vi "Teleop.vi"(10 "Match Info":T1={"Autonomous Elapsed Seconds"=0.0, "TeleOp Elapsed Seconds"=0.0, "Disabled Elapsed Seconds"=0.0, "Visited Autonomous"=FALSE, "Visited TeleOp"=FALSE, "Visited Disabled"=FALSE, "Autonomous Settings"={"Autonomous Style"=enum."Independent", "VI Refnum"=refnum}}, 11 "Call Context":T2) -> ()   [LabVIEW 2016]
doc: "This VI is called for each TeleOp packet received from the DS where the robot is not disabled. It is often used to read from the joysticks and update I/O or to update setpoints for timed control loops. It should complete and return within 20 milliseconds or it may miss DS packets."
uses:
  <vilib>/Rock Robotics/WPI/DriverStation/WPI_DriverStationDerivedRobotMode.ctl
  <vilib>/Rock Robotics/WPI/DriverStation/WPI_DriverStationMatch Info.ctl
  <vilib>/Rock Robotics/WPI/ThirdParty/CanMotor/TalonSRX/WPI_CANTalonSRX_APIFeedbackSelect.ctl
  <vilib>/Rock Robotics/WPI/ThirdParty/CanMotor/TalonSRX/WPI_CANTalonSRX_Params.ctl
  <vilib>/Rock Robotics/WPI/ThirdParty/CanMotor/TalonSRX/WPI_CANTalonSRX_APIControlMode.ctl
  <vilib>/Rock Robotics/WPI/Utilities/WPI_GetSetVariantRefNum.vi
panel:
  out "SensorPos (rotations)":dbl
  out "Motor output Plot":cluster{"Applied Throttle":dbl}(graph)
  out "Target Position (rotations)":dbl
  out "SensorRPM Velocity RPM":dbl
  in  "Ramp Rate":dbl
  in  "I Zone":dbl
  in  "F - Generally is zero for position-servo":dbl
  in  "D":dbl
  in  "I":dbl
  in  "P":dbl
  out "Applied Output":dbl
  out "Position Closed Loop Plots":cluster{dbl, "Sensor Velocity":dbl}(graph)
  # "Press and Hold Button1 to drive Talon directly.  Make sure sensor position moves in positive direction when Talon LEDs are green.\n\nMomentary press Button2 to activate Position closed-loop.  The gamepad y-axis is sampled once and scaled to provide a target set point.\n\nPress Button3 to \"zero\" the sensor position.\n\nPress Button4 to \"seed\" the Sensor position with the Absolute Position reported by the CTRE Magnetic Encoder."
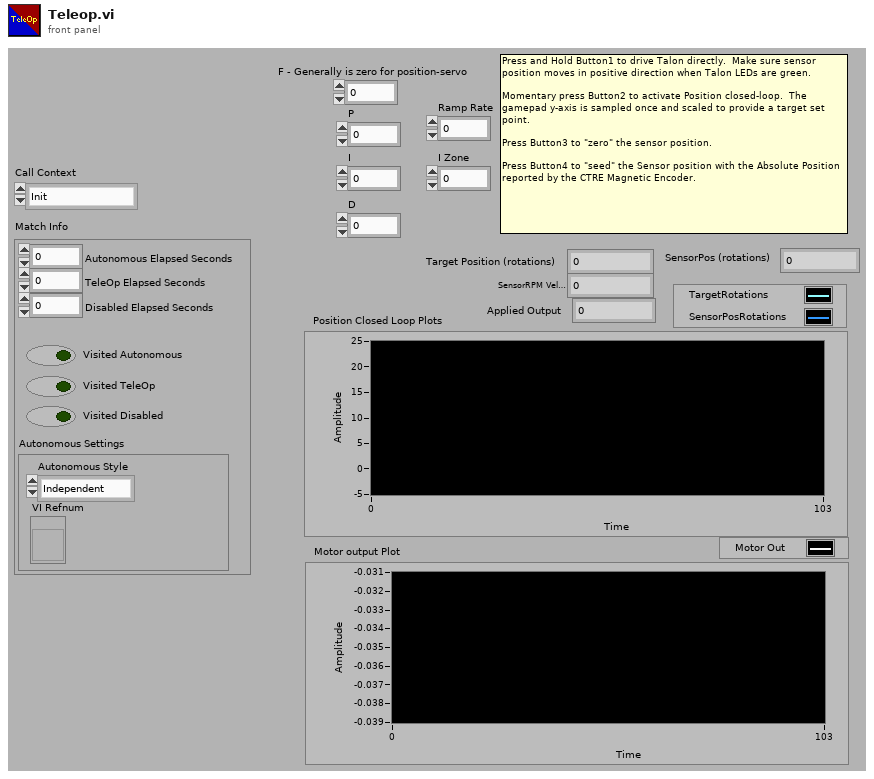
[diagram p1: front panel]
types:
  T1 = typedef "WPI_DriverStationMatch Info.ctl" = cluster{"Autonomous Elapsed Seconds":dbl, "TeleOp Elapsed Seconds":dbl, "Disabled Elapsed Seconds":dbl, "Visited Autonomous":bool, "Visited TeleOp":bool, "Visited Disabled":bool, "Autonomous Settings":cluster{"Autonomous Style":enum16{"Iterative", "Independent"}, "VI Refnum":refnum<vi>}}
  T2 = typedef "WPI_DriverStationDerivedRobotMode.ctl" = enum16{"Init", "Execute", "Stop"}
  T3 = typedef "WPI_CANTalonSRX_APIFeedbackSelect.ctl" = enum16{"Digital Quadrature Encoder", "Analog Potentiometer", "Analog Encoder", "Count on Quad-A (Rising-Edge)", "Count on Quad-A (Falling-Edge)", "CTR Magnetic Enc (Absolute)", "CTR Magnetic Enc (Relative)", "Pulse Width"}
  T4 = typedef "WPI_JoystickDevRef.ctl" = cluster{"Device":T5}
  T5 = typedef "WPI_JoystickDeviceEnum.ctl" = enum16{"USB 0", "USB 1", "USB 2", "USB 3", "USB 4", "USB 5"}
  T6 = typedef "WPI_MotorControlDeviceRef.ctl" = cluster{"DeviceStatus":errorcluster, "Type":T7, "PWM":cluster{"PWM Channel":T8, "DeadBand":T9}, "CAN":cluster{"Device Number":u8, "SetOutput VI Ref":variant, "GetOutput VI Ref":variant, "Enable VI Ref":variant, "Disable VI Ref":variant, "Data":variant}, "Invert":bool}
  T7 = typedef "WPI_MotorControlType.ctl" = enum16{"PWM", "CAN"}
  T8 = typedef "FPGA_DIOPWMChannel.ctl" = enum8{"PWM 0", "PWM 1", "PWM 2", "PWM 3", "PWM 4", "PWM 5", "PWM 6", "PWM 7", "PWM 8", "PWM 9", "PWM MXP 0", "PWM MXP 1", "PWM MXP 2", "PWM MXP 3", "PWM MXP 4", "PWM MXP 5", "PWM MXP 6", "PWM MXP 7", "PWM MXP 8", "PWM MXP 9", "Invalid"}
  T9 = typedef "WPI_PWMDeadband.ctl" = cluster{"Name":string, "maxPositivePwm":i32, "minPositivePwm":i32, "centerPwm":i32, "maxNegativePwm":i32, "minNegativePwm":i32, "angularRange":u16}
  T10 = typedef "WPI_CANTalonSRX_APIControlMode.ctl" = enum8{"Percent VBus", "Speed", "Position", "Slave", "Unchanged / Invalid", "Voltage Compensation", "Current", "Motion Profile", "Motion Magic"}
  T11 = typedef "WPI_CANTalonSRX_Params.ctl" = u8
  T12 = typedef "WPI_CANTalonSRX_GlobalStatus.ctl" = cluster{"Applied Throttle":dbl, "Module Enabled":bool, "CAN Error":errorcluster, "Closed Loop Error":dbl, "Forward Limit Switch Closed":bool, "Reverse Limit Switch Closed":bool, "Sensor Position":dbl, "Sensor Velocity":dbl, "Current":dbl, "Sticky Fault - Over Temp":bool, "Sticky Fault - Under Voltage":bool, "Sticky Fault - Forward Limit":bool, "Sticky Fault - Reverse Limit":bool, "Sticky Fault - Forward Soft Limit":bool, "Sticky Fault - Reverse Soft Limit":bool, "Brake is Enabled":bool, "Encoder Position":dbl, "Encoder Velocity":dbl, "Encoder Index Count":dbl, "Encoder A Pin State":bool, "Encoder B Pin State":bool, "Encoder Index Pin State":bool, "Analog In":dbl, "Analog In Velocity":dbl, "Temperature (C)":dbl, "Battery Voltage":dbl, "Control 5 Is Supported":bool, "Current Profile Slot Select":dbl, "Pos Div 8":bool, "Vel Div 4":bool, "Pulse Width Position":i32, "Pulse Width Velocity":i32, "Pulse Width Rise To Rise (us)":i32, "Pulse Width Rise To Fall (us)":i32, "Mot Prof Active Is Under Run":bool, "Mot Prof Active Has Under Run":bool, "Mot Prof Active Is Last":bool, "Mot Prof Active Velocity Only":bool, "Mot Prof Active Is Valid":bool, "Mot Prof Buffer Is Full":bool, "Mot Prof Active Profile Slot Select":i32, "Mot Prof NextID":i32, "Mot Prof Count":i32, "Mot Prof Active Velocity":dbl, "Mot Prof Active Position":dbl, "Mot Prof Output Enable":i32}
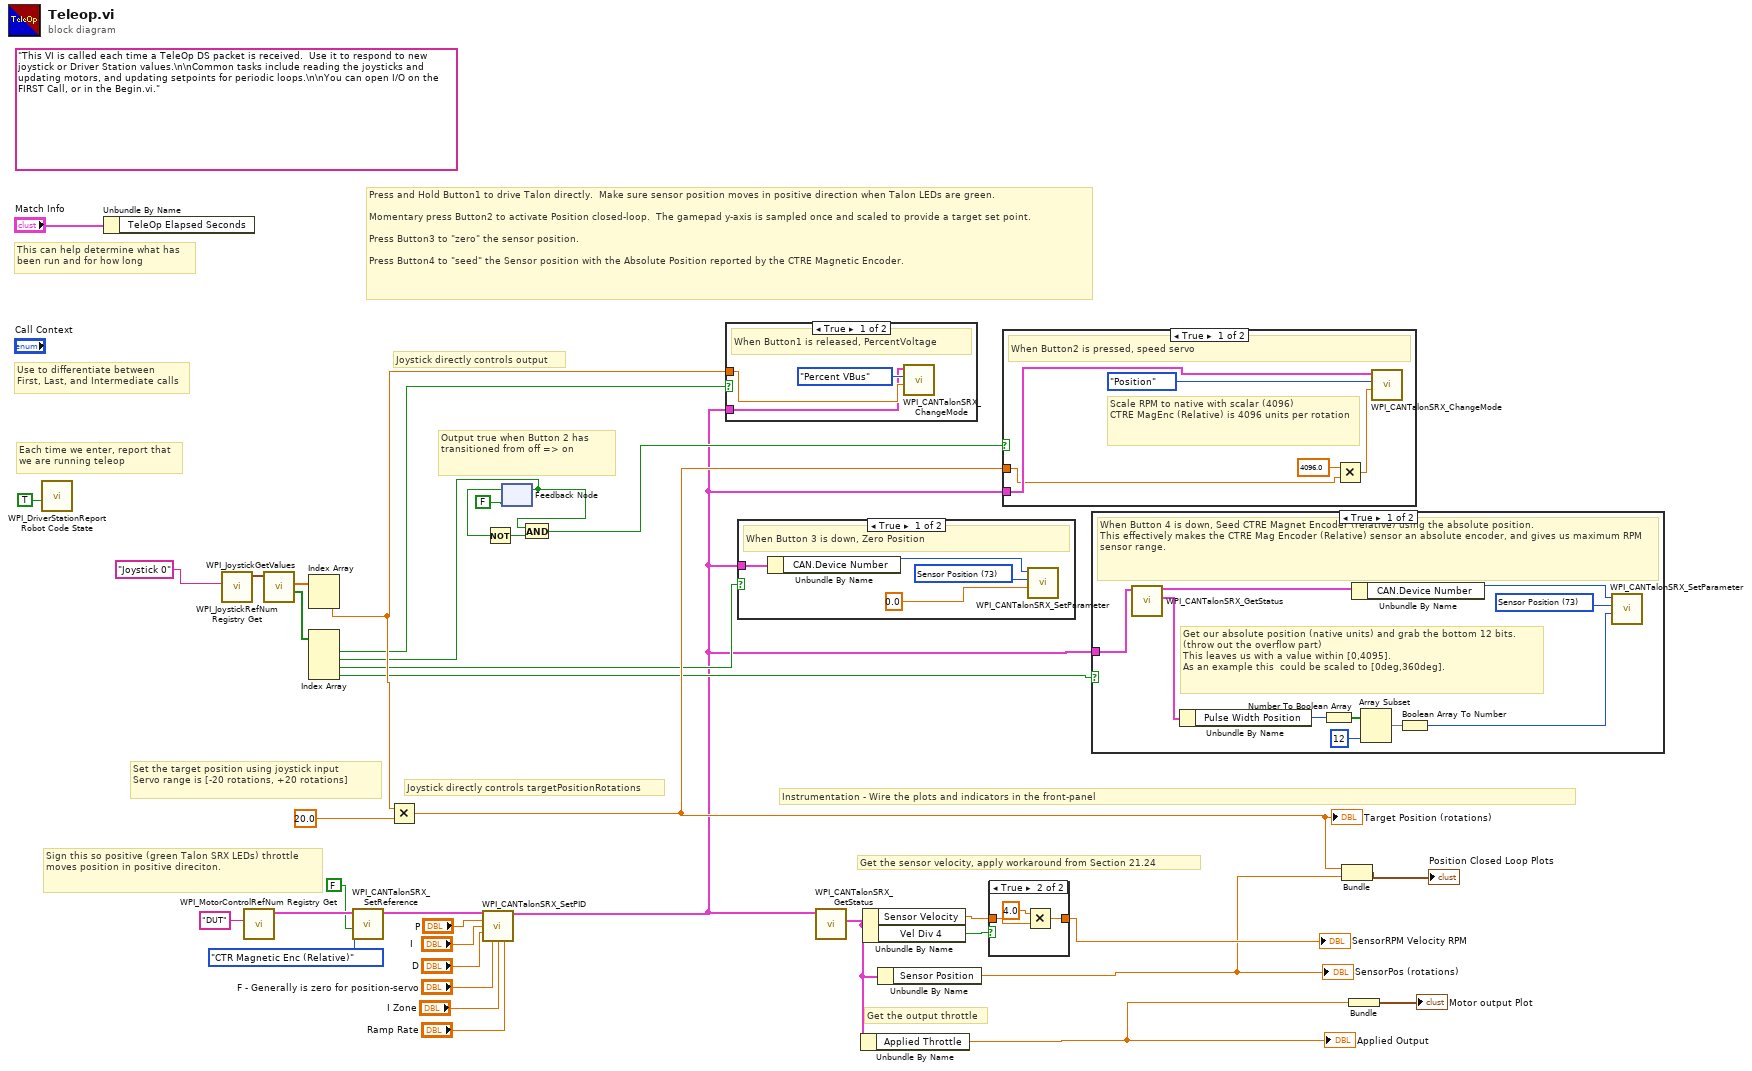
[diagram p0: block diagram]
diagram:
  (unwired) "This VI is called each time a TeleOp DS packet is received.  Use it to respond to new joystick or Driver Station values.\n\nCommon tasks include reading the joysticks and updating motors, and updating setpoints for periodic loops.\n\nYou can open I/O on the FIRST Call, or in the Begin.vi."
  # "Sign this so positive (green Talon SRX LEDs) throttle moves position in positive direciton."
  # "Instrumentation - Wire the plots and indicators in the front-panel"
  # "Output true when Button 2 has transitioned from off => on"
  # "Press and Hold Button1 to drive Talon directly.  Make sure sensor position moves in positive direction when Talon LEDs are green.\n\nMomentary press Button2 to activate Position closed-loop.  The gamepad y-axis is sampled once and scaled to provide a target set point.\n\nPress Button3 to \"zero\" the sensor position.\n\nPress Button4 to \"seed\" the Sensor position with the Absolute Position reported by the CTRE Magnetic Encoder."
  # "Get the output throttle"
  # "Get the sensor velocity, apply workaround from Section 21.24"
  # "Joystick directly controls targetPositionRotations"
  # "Joystick directly controls output"
  # "Set the target position using joystick input\nServo range is [-20 rotations, +20 rotations]"
  # "Each time we enter, report that\nwe are running teleop"
  # "Use to differentiate between\nFirst, Last, and Intermediate calls"
  # "This can help determine what has\nbeen run and for how long"
  n1 = call <vilib>:"WPI_DriverStationReport Robot Code State.vi"("TeleOp"=TRUE ("Autonomous")) -> ()  [unwired: 10 in, 1 out]
  n2 = Unbundle By Name("Match Info") -> ()  [unwired: 1 out]
  n3 = call <vilib>:"WPI_JoystickRefNum Registry Get.vi"("refnum name"="Joystick 0") -> ("JoystickDevRef"=w35:T4)  [unwired: 1 in, 9 out]
  n4 = call <vilib>:"WPI_MotorControlRefNum Registry Get.vi"("refnum name"="DUT") -> ("MotorControlDevRef"=w19:T6)  [unwired: 9 in, 1 out]
  n5 = call <vilib>:"WPI_JoystickGetValues.vi"("JoystickDevRef"=w35) -> ("Buttons"=w32:bool[], "Axes"=w33:dbl[])  [unwired: 6 in, 3 out]
  n6 = Index Array(array=w33) -> (element #2=w12:dbl)  [unwired: 2 in, 1 out]
  n7 = Index Array(array=w32) -> (element #1=w9:bool, element #2=w7:bool, element #3=w5:bool, element #4=w3:bool)  [unwired: 4 in]
  n8 = call <vilib>:"WPI_CANTalonSRX_SetReference.vi"("Reverse Feedback Sensor"=FALSE, "Feedback Reference"=WPI_CANTalonSRX_APIFeedbackSelect."CTR Magnetic Enc (Relative)", "CAN Talon SRX Ref"=w19) -> ("CAN Talon SRX Ref"=w18:T6)  [unwired: 7 in, 1 out]
  n9 = Multiply(x=w12, y=20.0) -> (x*y=w6:dbl)
  "Target Position (rotations)" <- w6
  n10 = call <vilib>:"WPI_CANTalonSRX_SetPID.vi"("CAN Talon SRX Ref"=w18, "P"="P", "I"="I", "D"="D", "F"="F - Generally is zero for position-servo", "I Zone"="I Zone", "Ramp Rate"="Ramp Rate") -> ("CAN Talon SRX Ref"=w1:T6)  [unwired: 7 in, 1 out]
  n11 = feedback-in #1(w7) -> ()
  n12 = feedback #1(FALSE) -> (w8:bool)
  n13 = Not(x=w8) -> (.not. x?=w10:bool)
  n14 = And(x=w7, y=w10) -> (x .and. y?=w2:bool)
  n15 = case shown="True" w9 {
    tunnel: w12 -> [w39 _]
    tunnel: w1 -> [w38 _]
    frame True {
      # "When Button1 is released, PercentVoltage"
      n16 = call <vilib>:"WPI_CANTalonSRX_ChangeMode.vi"("Output"=w39, "Control Mode"=WPI_CANTalonSRX_APIControlMode."Percent VBus", "CAN Talon SRX Ref"=w38) -> ()  [unwired: 7 in, 2 out]
    }
    frame False {
    }
  }
  n17 = case shown="True" w5 {
    tunnel: w1 -> [w41 _]
    frame True {
      w44 = T11 73 items=["Slot 0 - P"=1, "Slot 0 - I"=2, "Slot 0 - D"=3, "Slot 0 - F"=4, "Slot 0 - I Zone"=5, "Slot 0 - Ramp Rate"=6, "Slot 1 - P"=11, "Slot 1 - I"=12, "Slot 1 - D"=13, "Slot 1 - F"=14, "Slot 1 - I Zone"=15, "Slot 1 - Ramp Rate"=16, "Soft Limit - Forward"=21, "Soft Limit - Reverse"=22, "Soft Limit - Forward Enable"=23, "Soft Limit - Reverse Enable"=24, "On Boot - Brake Mode"=31, "On Boot - Limit Normally Closed - Forward"=32, "On Boot - Limit Normally Closed - Reverse"=33, "On Boot - Limit Disabled - Forward"=34, "On Boot - Limit Disabled - Reverse"=35, "Fault - Over Temp"=41, "Fault - Under Voltage"=42, "Fault - Forward Limit"=43, "Fault - Reverse Limit"=44, "Fault - Hardware Failure"=45, "Fault - Forward Soft Limit"=46, "Fault - Reverse Soft Limit"=47, "Sticky Fault - Over Temp"=48, "Sticky Fault - Under Voltage"=49, "Sticky Fault - Forward Limit"=50, "Sticky Fault - Reverse Limit"=51, "Sticky Fault - Forward Soft Limit"=52, "Sticky Fault - Reverse Soft Limit"=53, "Applied Throttle"=61, "Closed-Loop Error"=62, "Select Feedback Device"=63, "Reverse Closed-Loop Output"=64, "Mode Select"=65, "Profile Slot Select"=66, "Ramp Throttle"=67, "Reverse Feedback Sensor"=68, "Limit Switch Enabled"=69, "Limit Switch Closed - Forward"=70, "Limit Switch Closed - Reverse"=71, "Sensor Position"=73, "Sensor Velocity"=74, "Current"=75, "Brake is Enabled"=76, "Encoder Position"=77, "Encoder Velocity"=78, "Encoder Index Rise Events"=79, "Encoder A Pin State"=80, "Encoder B Pin State"=81, "Encoder Index Pin State"=82, "Analog In with Overflow"=83, "Analog In Velocity"=84, "Temperature"=85, "Battery Voltage"=86, "Reset Count"=87, "Reset Flags"=88, "Firmware Version"=89, "Settings Changed"=90, "Quad Filter Enable"=91, "Ignore Disable Broadcast"=92, "I Accumulator"=93, "Status 1 Frame Rate Ms"=94, "Status 2 Frame Rate Ms"=95, "Status 3 Frame Rate Ms"=96, "Status 4 Frame Rate Ms"=97, "Status 6 Frame Rate Ms"=98, "Status 7 Frame Rate Ms"=99, "Enable Index Pin Clear Position"=100, "Peak Positive Output"=104, "Nominal Positive Output"=105, "Peak Negative Output"=106, "Nominal Negative Output"=107, "Quad Index Pin Polarity"=108, "Status 8 Frame Rate Ms"=109, "Allow Position Overflow"=110, "Slot 0 - Allowable Closed-Loop Error"=111, "Number Potentiometer Turns"=112, "Encoder Codes Per Rev"=113, "Pulse Width Decoded Position"=114, "Analog Position"=115, "Voltage Compensation Rate (V/s)"=116, "Slot 1 - Allowable Closed-Loop Error"=117, "Motion Profile Has Underrun Err"=119] ("Parameter")
      # "When Button 3 is down, Zero Position"
      n18 = Unbundle By Name(w41) -> ("CAN.Device Number"=w43:u8)
      n19 = call <vilib>:"WPI_CANTalonSRX_SetParameter.vi"("Value"=0.0, "Parameter"=w44, "Device ID (0)"=w43) -> ()  [unwired: 7 in, 2 out]
    }
    frame False {
    }
  }
  n20 = call <vilib>:"WPI_CANTalonSRX_GetStatus.vi"("CAN Talon SRX Ref"=w1) -> ("Talon SRX Status"=w16:T12)  [unwired: 8 in, 2 out]
  n21 = Unbundle By Name(w16) -> ("Applied Throttle"=w14:dbl)
  "Applied Output" <- w14
  n22 = Unbundle By Name(w16) -> ("Sensor Velocity"=w22:dbl, "Vel Div 4"=w21:bool)
  n23 = Unbundle By Name(w16) -> ("Sensor Position"=w13:dbl)
  "SensorPos (rotations)" <- w13
  n24 = case shown="True" w21 {
    tunnel: [w45 w47] -> w20
    tunnel: w22 -> [w45 w46]
    frame False {
    }
    frame True {
      n25 = Multiply(x=4.0, y=w46) -> (x*y=w47:dbl)
    }
  }
  "SensorRPM Velocity RPM" <- w20
  n26 = case shown="True" w2 {
    tunnel: w6 -> [w49 _]
    tunnel: w1 -> [w50 _]
    frame True {
      # "Scale RPM to native with scalar (4096)\nCTRE MagEnc (Relative) is 4096 units per rotation"
      # "When Button2 is pressed, speed servo"
      n27 = Multiply(x=4096.0, y=w49) -> (x*y=w52:dbl)
      n28 = call <vilib>:"WPI_CANTalonSRX_ChangeMode.vi"("Output"=w52, "Control Mode"=WPI_CANTalonSRX_APIControlMode."Position", "CAN Talon SRX Ref"=w50) -> ()  [unwired: 7 in, 2 out]
    }
    frame False {
    }
  }
  n29 = case shown="True" w3 {
    tunnel: w1 -> [w54 _]
    frame True {
      w63 = T11 73 items=["Slot 0 - P"=1, "Slot 0 - I"=2, "Slot 0 - D"=3, "Slot 0 - F"=4, "Slot 0 - I Zone"=5, "Slot 0 - Ramp Rate"=6, "Slot 1 - P"=11, "Slot 1 - I"=12, "Slot 1 - D"=13, "Slot 1 - F"=14, "Slot 1 - I Zone"=15, "Slot 1 - Ramp Rate"=16, "Soft Limit - Forward"=21, "Soft Limit - Reverse"=22, "Soft Limit - Forward Enable"=23, "Soft Limit - Reverse Enable"=24, "On Boot - Brake Mode"=31, "On Boot - Limit Normally Closed - Forward"=32, "On Boot - Limit Normally Closed - Reverse"=33, "On Boot - Limit Disabled - Forward"=34, "On Boot - Limit Disabled - Reverse"=35, "Fault - Over Temp"=41, "Fault - Under Voltage"=42, "Fault - Forward Limit"=43, "Fault - Reverse Limit"=44, "Fault - Hardware Failure"=45, "Fault - Forward Soft Limit"=46, "Fault - Reverse Soft Limit"=47, "Sticky Fault - Over Temp"=48, "Sticky Fault - Under Voltage"=49, "Sticky Fault - Forward Limit"=50, "Sticky Fault - Reverse Limit"=51, "Sticky Fault - Forward Soft Limit"=52, "Sticky Fault - Reverse Soft Limit"=53, "Applied Throttle"=61, "Closed-Loop Error"=62, "Select Feedback Device"=63, "Reverse Closed-Loop Output"=64, "Mode Select"=65, "Profile Slot Select"=66, "Ramp Throttle"=67, "Reverse Feedback Sensor"=68, "Limit Switch Enabled"=69, "Limit Switch Closed - Forward"=70, "Limit Switch Closed - Reverse"=71, "Sensor Position"=73, "Sensor Velocity"=74, "Current"=75, "Brake is Enabled"=76, "Encoder Position"=77, "Encoder Velocity"=78, "Encoder Index Rise Events"=79, "Encoder A Pin State"=80, "Encoder B Pin State"=81, "Encoder Index Pin State"=82, "Analog In with Overflow"=83, "Analog In Velocity"=84, "Temperature"=85, "Battery Voltage"=86, "Reset Count"=87, "Reset Flags"=88, "Firmware Version"=89, "Settings Changed"=90, "Quad Filter Enable"=91, "Ignore Disable Broadcast"=92, "I Accumulator"=93, "Status 1 Frame Rate Ms"=94, "Status 2 Frame Rate Ms"=95, "Status 3 Frame Rate Ms"=96, "Status 4 Frame Rate Ms"=97, "Status 6 Frame Rate Ms"=98, "Status 7 Frame Rate Ms"=99, "Enable Index Pin Clear Position"=100, "Peak Positive Output"=104, "Nominal Positive Output"=105, "Peak Negative Output"=106, "Nominal Negative Output"=107, "Quad Index Pin Polarity"=108, "Status 8 Frame Rate Ms"=109, "Allow Position Overflow"=110, "Slot 0 - Allowable Closed-Loop Error"=111, "Number Potentiometer Turns"=112, "Encoder Codes Per Rev"=113, "Pulse Width Decoded Position"=114, "Analog Position"=115, "Voltage Compensation Rate (V/s)"=116, "Slot 1 - Allowable Closed-Loop Error"=117, "Motion Profile Has Underrun Err"=119] ("Parameter")
      # "Get our absolute position (native units) and grab the bottom 12 bits. (throw out the overflow part)  \nThis leaves us with a value within [0,4095]. \nAs an example this  could be scaled to [0deg,360deg]."
      # "When Button 4 is down, Seed CTRE Magnet Encoder (relative) using the absolute position.\nThis effectively makes the CTRE Mag Encoder (Relative) sensor an absolute encoder, and gives us maximum RPM sensor range."
      n30 = call <vilib>:"WPI_CANTalonSRX_GetStatus.vi"("CAN Talon SRX Ref"=w54) -> ("Talon SRX Status"=w61:T12, "CAN Talon SRX Ref"=w60:T6)  [unwired: 8 in, 1 out]
      n31 = Unbundle By Name(w61) -> ("Pulse Width Position"=w59:i32)
      n32 = Number To Boolean Array(number=w59) -> (Boolean array=w57:bool[])
      n33 = Unbundle By Name(w60) -> ("CAN.Device Number"=w62:u8)
      n34 = Array Subset(array=w57, length=12 ("index")) -> (w56:bool[])  [unwired: 1 in]
      n35 = Boolean Array To Number(Boolean array=w56) -> (number=w55:u32)
      n36 = call <vilib>:"WPI_CANTalonSRX_SetParameter.vi"("Value"=w55, "Parameter"=w63, "Device ID (0)"=w62) -> ()  [unwired: 7 in, 2 out]
    }
    frame False {
    }
  }
  n37 = Bundle(w6, "Sensor Position"=w13) -> (→"Position Closed Loop Plots":cluster{dbl, "Sensor Position":dbl})  [unwired: 1 in]
  n38 = Bundle("Applied Throttle"=w14) -> (→"Motor output Plot":cluster{"Applied Throttle":dbl})  [unwired: 1 in]
